vi "emi_Pane Background.vi"(0 "Pane Refnum":refnum<vi>, 1 "Width(Screen)":i32=-1, 2 "Height(Screen)":i32=-1, 3 "Dark(Black)":u32(colorbox), 4 "Light(White)":u32(colorbox)=16448250, 5 "error in":errorcluster, 6 "Graphic Type(FlatColor)":T1) -> (14 "Pane Refnum out":refnum<vi>, 19 "error out":errorcluster)   [LabVIEW 2011]
doc: "Set the background graphic for a VI frontpanel pane. \nNote that with and height must be bigger then the largest size for the pane. If left blank, a background the size of the screen is generated.\n\nOn error: No action performed"
uses:
  0 - General/Graphix/Private/emi_List Of Graphix.ctl
  <vilib>/picture/picture.llb/imagedata.ctl
  0 - General/Graphix/emi_BW 8Bit image to Linear DuoTone.vi
  0 - General/Graphix/emi_Tile Gradient Image.vi
  <vilib>/picture/picture.llb/Draw Flattened Pixmap.vi
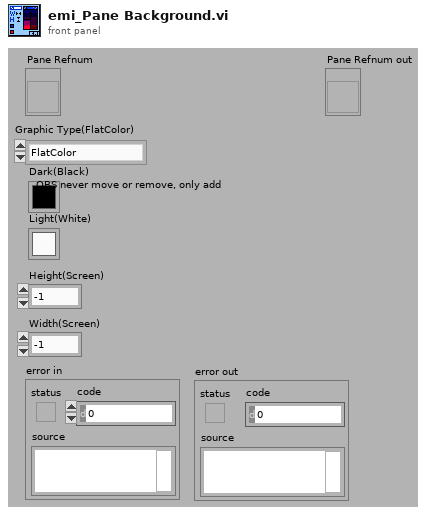
[diagram p1: front panel]
types:
  T1 = typedef "emi_List Of Graphix.ctl" = enum16{"FlatColor", "SharpGrad", "ShallowGrad", "GlasGradBord", "GlasGrad", "GlasGradBord 2"}
  T2 = typedef "imagedata.ctl" = cluster{"image type":i32, "image depth":i32, "image":u8[], "mask":u8[], "colors":u32[], "Rectangle":cluster{"left":i16, "top":i16, "right":i16, "bottom":i16}}
  T3 = typedef "LVRectTypeDef.ctl" = cluster{"left":i16, "top":i16, "right":i16, "bottom":i16}
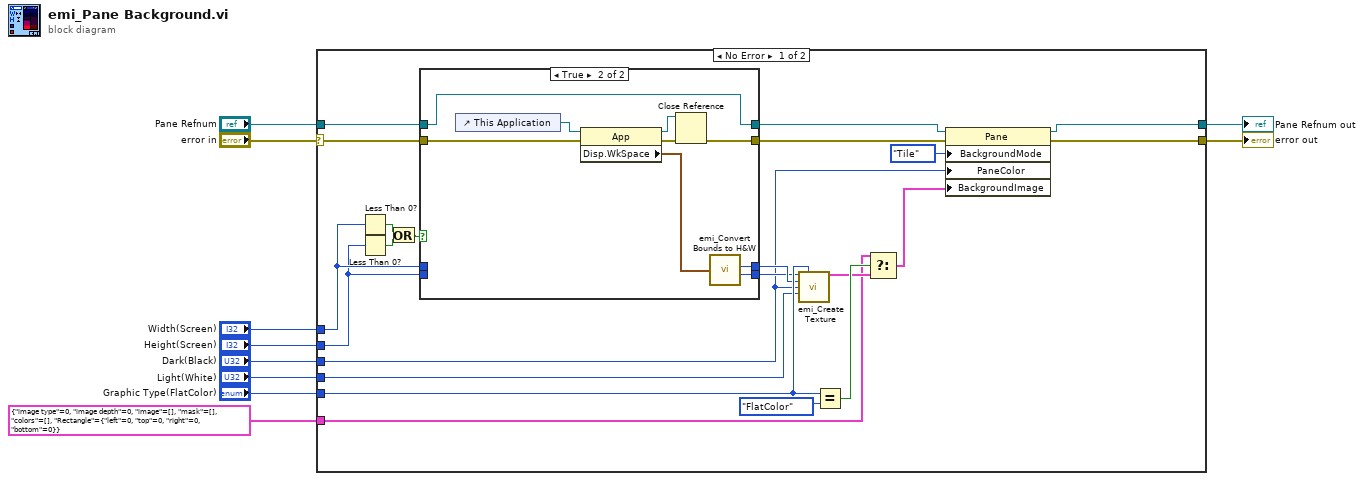
[diagram p0: block diagram]
diagram:
  n1 = case shown="No Error" "error in" {
    selector: "error in" -> [w22 w47]
    tunnel: "Graphic Type(FlatColor)" -> [w31 _]
    tunnel: T2 {"image type"=0, "image depth"=0, "image"=[], "mask"=[], "colors"=[], "Rectangle"={"left"=0, "top"=0, "right"=0, "bottom"=0}} ("Image Data Out") -> [w16 _]
    tunnel: "Pane Refnum" -> [w26 w46]
    tunnel: "Width(Screen)" -> [w25 _]
    tunnel: "Height(Screen)" -> [w24 _]
    tunnel: "Dark(Black)" -> [w18 _]
    tunnel: "Light(White)" -> [w30 _]
    tunnel: [w11 w47] -> w2
    tunnel: [w13 w46] -> w1
    frame No Error {
      n2 = Less Than 0?(x=w25) -> (x < 0?=w27:bool)
      n3 = Less Than 0?(x=w24) -> (x < 0?=w28:bool)
      n4 = Or(x=w27, y=w28) -> (x .or. y?=w23:bool)
      n5 = case shown="True" w23 {
        tunnel: w26 -> [w36 w37]
        tunnel: [w36 w37] -> w14
        tunnel: w22 -> [w35 w44]
        tunnel: [w35 w39] -> w12
        tunnel: w25 -> [w34 _]
        tunnel: [w34 w42] -> w21
        tunnel: w24 -> [w33 _]
        tunnel: [w33 w41] -> w20
        frame False {
        }
        frame True {
          n6 = control-ref of="This Application"() -> (w45:refnum<vi>)
          n7 = property class="App"(reference=w45, error in=w44) -> (reference out=w38:refnum<vi>, error out=w40:errorcluster, "Disp.WkSpace"=w43:T3)
          n8 = Close Reference(reference=w38, error in (no error)=w40) -> (error out=w39:errorcluster)
          n9 = call "emi_Convert Bounds to H&W.vi"("Bounds"=w43) -> ("Width"=w42:i32, "Height"=w41:i32)  [unwired: 6 in]
        }
      }
      n10 = call "emi_Create Texture.vi"("Height(600)"=w20, "Graphic Type(Flat Color)"=w31, "Width(400)"=w21, "Dark(Black)"=w18, "Light(White)"=w30) -> ("Image Data Out"=w17:T2)  [unwired: 8 in, 2 out]
      n11 = Equal?(x=w31, y=emi_List_Of_Graphix."FlatColor" ("Graphic Type")) -> (x = y?=w29:bool)
      n12 = Select(t=w16, s=w29, f=w17) -> (s? t:f=w15:T2)
      n13 = property class="Pane"(reference=w14, error in=w12, "BackgroundMode"=enum16{"Stretch", "Center", "Tile"}."Tile" ("Background Mode"), "PaneColor"=w18, "BackgroundImage"=w15) -> (reference out=w13:refnum<vi>, error out=w11:errorcluster)
    }
    frame Error {
    }
  }
  "error out" <- w2
  "Pane Refnum out" <- w1
